vi "数值（I16）至布尔数组.vi"(11 "Num":i16) -> (3 "Boolean":bool[](array[boolean]))   [LabVIEW 2012]
doc: "Converts a single I32 into an array of digits, in order of increasing significance. If the input number is negative, the most significant digit (last element of the array) is also negative. All other digits are always non-negative. By default, the output digits are the digits used to represent the number in base 10, though the base can be changed. For example, the binary representation can be obtained by wiring the value 2 to the Base input. Note that Base is coerced to a minimum value of 2.\n\nAs long as no coersion is required, the original number can be recreated as\nN = Digits[0] * Base^0 + Digits[1] * Base^1 + Digits[2] * Base^2 + ... + Digits[n] * Base^n\n\nFreeware from Moore Good Ideas, www.mooregoodideas.com. Do not remove this line."
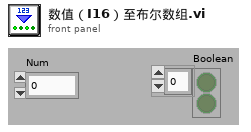
[diagram p1: front panel]
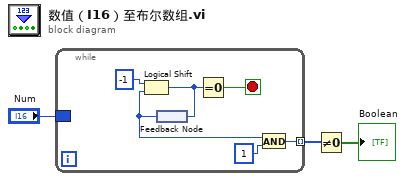
[diagram p0: block diagram]
diagram:
  n1 = while {
    tunnel: [w6] -> w3 mode=indexing
    border: "Num" -> [_]
    stop <- w8 stop-if-true
    n2 = feedback #1() -> (w5:i16)
    n3 = Logical Shift(y=i8 -1, x=w5) -> (x << y=w4:i16)
    n4 = feedback-in #1(w4) -> ()
    n5 = Equal To 0?(x=w4) -> (x = 0?=w8:bool)
    n6 = And(x=w5, y=i16 1) -> (x .and. y?=w6:i16)
  }
  n7 = Not Equal To 0?(x=w3) -> (x != 0?=→"Boolean":bool[])
